vi "Deserialize Data Frame.vi"(8 "error in (no error)":errorcluster, 9 "Batch Size":u64, 10 "FFT Size":u64, 11 "Serial Data In":refnum<class "1D Array s16.lvclass">) -> (0 "error out":errorcluster, 3 "Deserialized Data Out":refnum<class "3D Array s16.lvclass">)   [LabVIEW 2020, in "GPU FFT Calculator.lvlib" / "GPU FFT Calculator.lvclass"]
uses:
  GPU FFT Calculator.lvclass
  <vilib>/Natan Biesmans/G2CPU GPU and CPU HPC Toolkit/G2CPU Libraries/Arrays/3DArray/s16/3D Array s16.lvclass
  C:/Program Files/National Instruments/LabVIEW 2026/vi.lib/Natan Biesmans/G2CPU GPU and CPU HPC Toolkit/G2CPU Libraries/Arrays/Array/Array Prototype.lvclass
  <vilib>/Natan Biesmans/G2CPU GPU and CPU HPC Toolkit/G2CPU Libraries/Arrays/1DArray/s16/1D Array s16.lvclass
  <vilib>/Natan Biesmans/G2CPU GPU and CPU HPC Toolkit/G2CPU Libraries/Arrays/Array/Array Prototype.lvclass/Array Prototype.ctl
  032e556b-7b54-4525-89b0-52f51dab6dbd.vi
  94fe28fa-c578-4db0-8d5c-99b9ccb733d5.vi
  <vilib>/Natan Biesmans/G2CPU GPU and CPU HPC Toolkit/G2CPU Libraries/Arrays/Array/G2CPU Get Array Pointer.vi
  032e556b-7b54-4525-89b0-52f51dab6dbd.vi/a407d5fa-ce17-4a97-bfa3-b4ade1da9bb5.vi
  032e556b-7b54-4525-89b0-52f51dab6dbd.vi/e0916498-1f24-4399-b470-92cd1c4905cf.vi
  032e556b-7b54-4525-89b0-52f51dab6dbd.vi/8ad42d3e-cbfb-439f-ab0e-c2c37a880530.vi
  032e556b-7b54-4525-89b0-52f51dab6dbd.vi/f0a659a8-d4f9-4e22-9e69-2d739819b076.vi
  94fe28fa-c578-4db0-8d5c-99b9ccb733d5.vi/922c8ee7-4bf3-46f2-9490-f19464352921.vi
  94fe28fa-c578-4db0-8d5c-99b9ccb733d5.vi/98720ac4-ce2f-4a3d-809d-44a551af1506.vi
  94fe28fa-c578-4db0-8d5c-99b9ccb733d5.vi/4a0c74eb-d4af-4e7d-9862-c2f0a120418a.vi
  <vilib>/Natan Biesmans/G2CPU GPU and CPU HPC Toolkit/ArrayFire Driver/VIs/moddims.vi
  <vilib>/Natan Biesmans/G2CPU GPU and CPU HPC Toolkit/G2CPU Libraries/Arrays/Array/G2CPU Set Array Pointer.vi
  <vilib>/Natan Biesmans/G2CPU GPU and CPU HPC Toolkit/ArrayFire Driver/VIs/reorder.vi
  <vilib>/Natan Biesmans/G2CPU GPU and CPU HPC Toolkit/G2CPU Libraries/Arrays/Array/Array Prototype.lvclass
  <vilib>/Natan Biesmans/G2CPU GPU and CPU HPC Toolkit/G2CPU Libraries/Arrays/DataTypes/I16/s16.lvclass
  <vilib>/Natan Biesmans/G2CPU GPU and CPU HPC Toolkit/G2CPU Libraries/Arrays/1DArray/1D Array Prototype.lvclass
  <vilib>/Natan Biesmans/G2CPU GPU and CPU HPC Toolkit/G2CPU Libraries/Arrays/3DArray/3D Array Prototype.lvclass
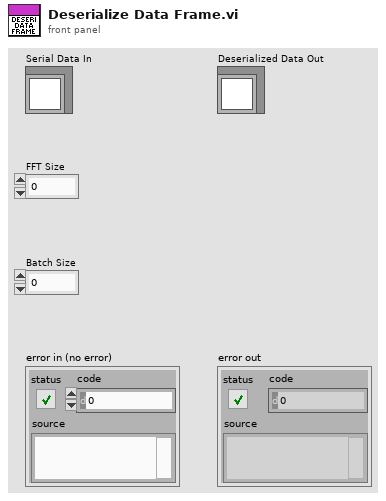
[diagram p1: front panel]
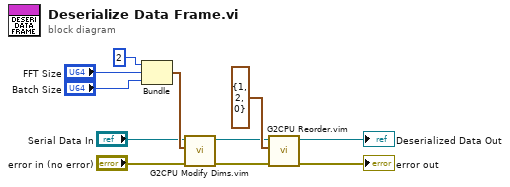
[diagram p0: block diagram]
diagram:
  n1 = Bundle(u64 2, "FFT Size"="FFT Size", "Batch Size"="Batch Size") -> (w6:cluster{u64, "FFT Size":u64, "Batch Size":u64})  [unwired: 1 in]
  n2 = call "G2CPU Modify Dims.vim"("error in (no error)"="error in (no error)", "dims"=w6, "Array In"="Serial Data In") -> ("error out"=w8:errorcluster, "Array out"=w7:refnum<class "3D Array s16.lvclass">)  [unwired: 7 in]
  n3 = call "G2CPU Reorder.vim"("error in (no error)"=w8, "Dim reorder"=cluster{"Dim 0":u64, "Dim 1":u64, "Dim 2":u64} {"Dim 0"=1, "Dim 1"=2, "Dim 2"=0}, "Array In"=w7) -> ("error out"=→"error out":errorcluster, "Array out"=→"Deserialized Data Out":refnum<class "3D Array s16.lvclass">)  [unwired: 7 in]
